vi "bloc_codage.vi"(9 "Array in":dbl[](array[numeric])) -> (1 "output bit stream":i8[](array[numeric]), 2 "sortie codeur convolutif":string, 3 "sortie générateur":string)   [LabVIEW 2018]
uses:
  <vilib>/addons/Modulation/niDMT.lvlib
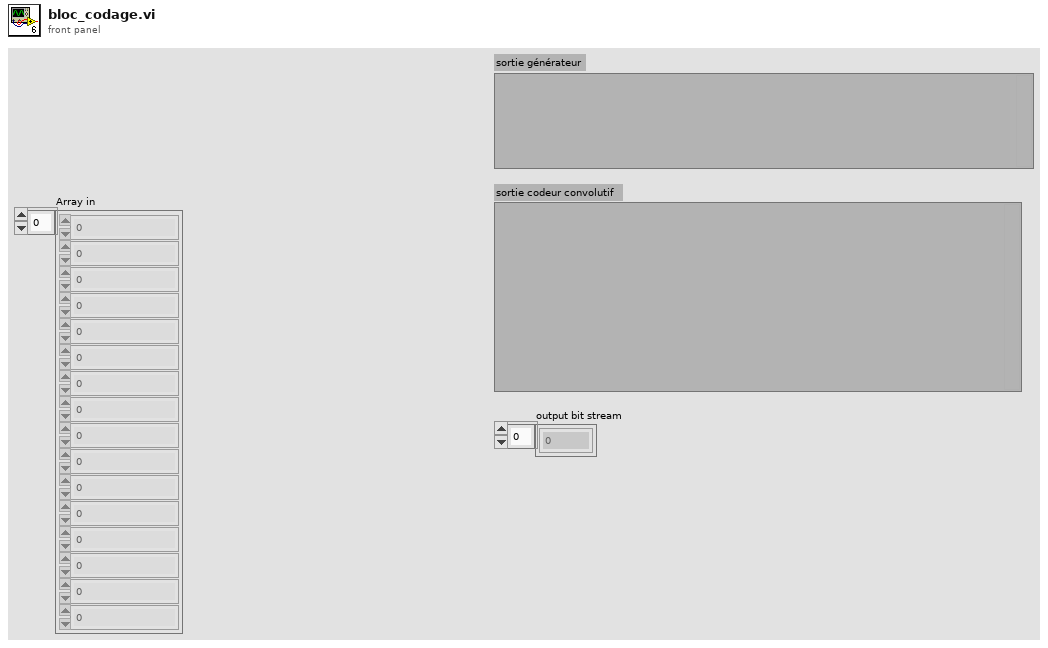
[diagram p1: front panel]
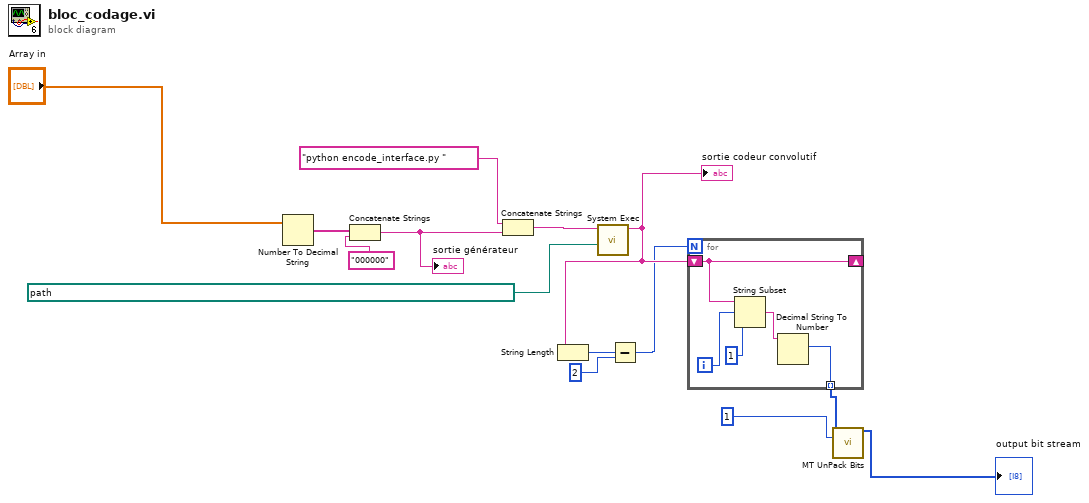
[diagram p0: block diagram]
diagram:
  n1 = Number To Decimal String(number="Array in") -> (decimal integer string=w13:string[])  [unwired: 1 in]
  n2 = Concatenate Strings(w13, "000000") -> (w11:string)
  "sortie générateur" <- w11
  n3 = Concatenate Strings("python encode_interface.py ", w11) -> (w10:string)
  n4 = call <vilib>:"System Exec.vi"("working directory"=path "C:/Users/pc-labview/Desktop/Levi/Turbo-Codes/Implémentation perso Python/BCJR_OO", "command line"=w10) -> ("standard output"=w8:string)  [unwired: 4 in, 5 out]
  "sortie codeur convolutif" <- w8
  n5 = String Length(string=w8) -> (length=w4:i32)
  n6 = Subtract(x=w4, y=2) -> (x-y=w5:i32)
  n7 = for {
    N: w5 -> [_]
    tunnel: [w16] -> w6 mode=indexing
    shift-right: [w15] -> _
    shift-left: w8 -> [w15]
    i -> [w19]
    n8 = String Subset(string=w15, offset (0)=w19, length (rest)=1) -> (substring=w17:string)
    n9 = Decimal String To Number(string=w17) -> (number=w16:i32)  [unwired: 2 in, 1 out]
  }
  n10 = call <vilib>:"MT UnPack Bits.vi"("input integers"=w6, "bits per integer"=1) -> ("output bit stream"=→"output bit stream":i8[])  [unwired: 12 in, 1 out]
